vi "AO Regs Group UI.vi"(8 "error in (no error)":errorcluster, 11 "Node Ptr":T2 format="%.0x") -> (0 "error out":errorcluster)   [LabVIEW 2021, in "Modbus Master System Explorer.lvlib"]
uses:
  Modbus Master System Explorer.lvlib
  <vilib>/NI VeriStand/Custom Device API/Custom Device Item Ref.ctl
  SubVIs/Conflict Table.ctl
  SubVIs/Modbus Type.ctl
  Shared/Controls/Data Model/Mapping.ctl
  Shared/Controls/Data Model/DataType.ctl
  <vilib>/NI VeriStand/Custom Device API/Custom Device API.lvlib
  <vilib>/NI VeriStand/Custom Device Tools/Custom Device Utility Library/Custom Device Utility Library.lvlib
  Shared/Modbus Master Shared.lvlib
panel:
  in  "Delete Multiple":bool
  in  "Add One":bool
  in  "Bulk Add":bool
  out "Conflicting Holding Register Mappings":T1
  in  "Header":cluster{"Section Name":string}={"Section Name"="Holding Register Group Settings"}
  in  "Description":string
  in  "Name":string
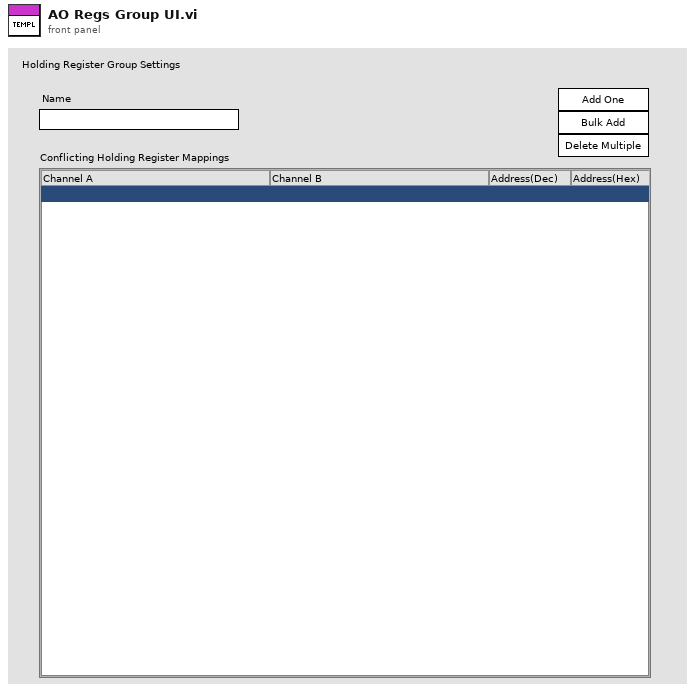
[diagram p1: front panel]
types:
  T1 = typedef "Modbus Master System Explorer.lvlib/Conflict Table.ctl" = i32
  T2 = typedef "Custom Device API.lvlib/Custom Device Item Ref.ctl" = u64
  T3 = typedef "Modbus Master Shared.lvlib/Modbus Type.ctl" = enum16{"Coil", "Discrete Input", "Holding Register", "Input Register"}
  T4 = typedef "Custom Device API.lvlib/Custom Device Item Info.ctl" = cluster{"Name":string, "Is Channel":bool, "GUID":string, "Is Waveform":bool}
  T5 = cluster{"Name":string, "Name":string, "Mapping":u16}[]
  T6 = typedef "Modbus Master Shared.lvlib/Mapping.ctl" = cluster{"DataType":T7, "Unit ID":u8, "Starting Address":u16, "Sub-Index (Bool)":u16, "VS Reference":T2}
  T7 = typedef "Modbus Master Shared.lvlib/DataType.ctl" = enum16{"Double", "Single", "I64", "I32", "I16", "I8", "U64", "U32", "U16", "U8", "Boolean"}
  T8 = typedef "Custom Device API.lvlib/Custom Device Commands.ctl" = enum16{"Default", "Item renamed", "Shutdown", "Dynamic button pressed"}
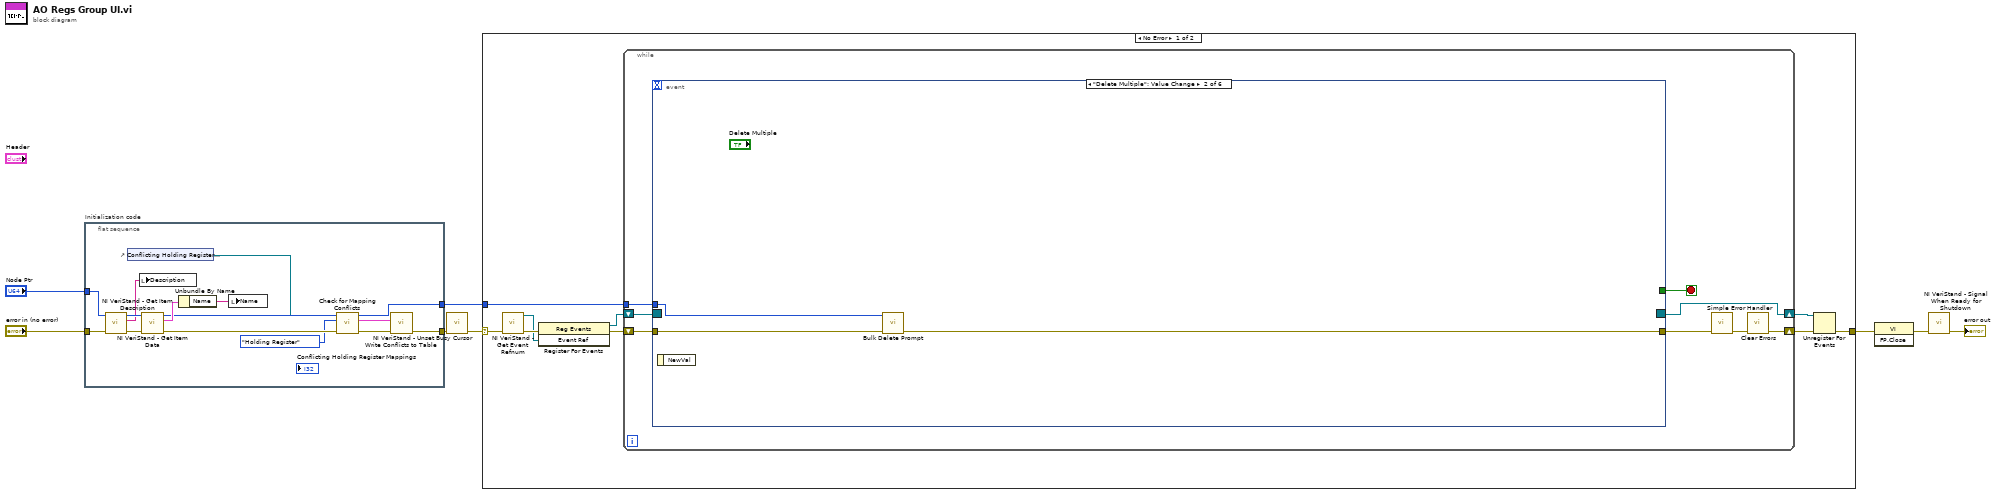
[diagram p0: block diagram]
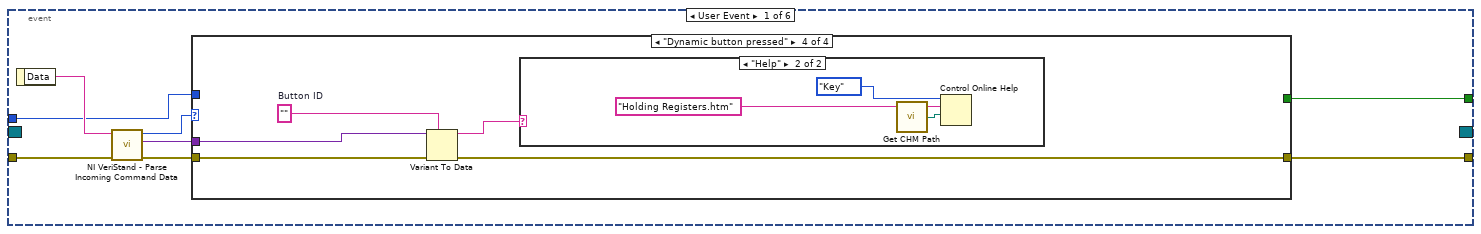
[diagram p2: hidden frame]
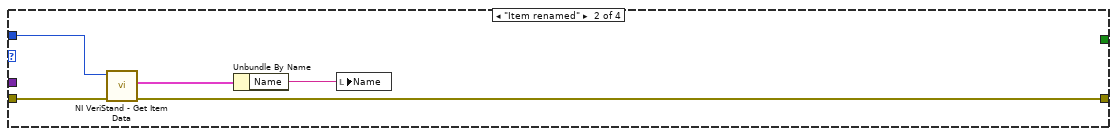
[diagram p4: hidden frame]
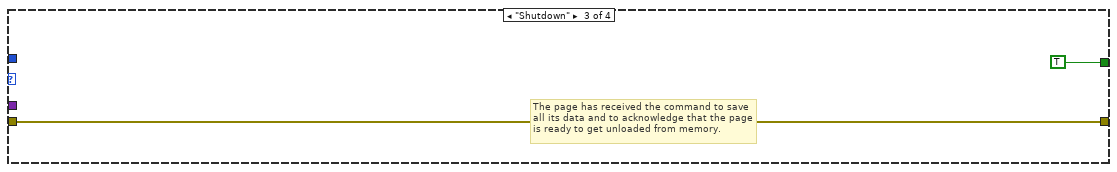
[diagram p5: hidden frame]
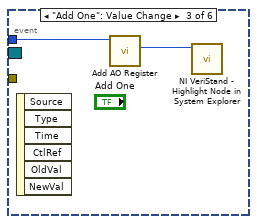
[diagram p7: hidden frame]
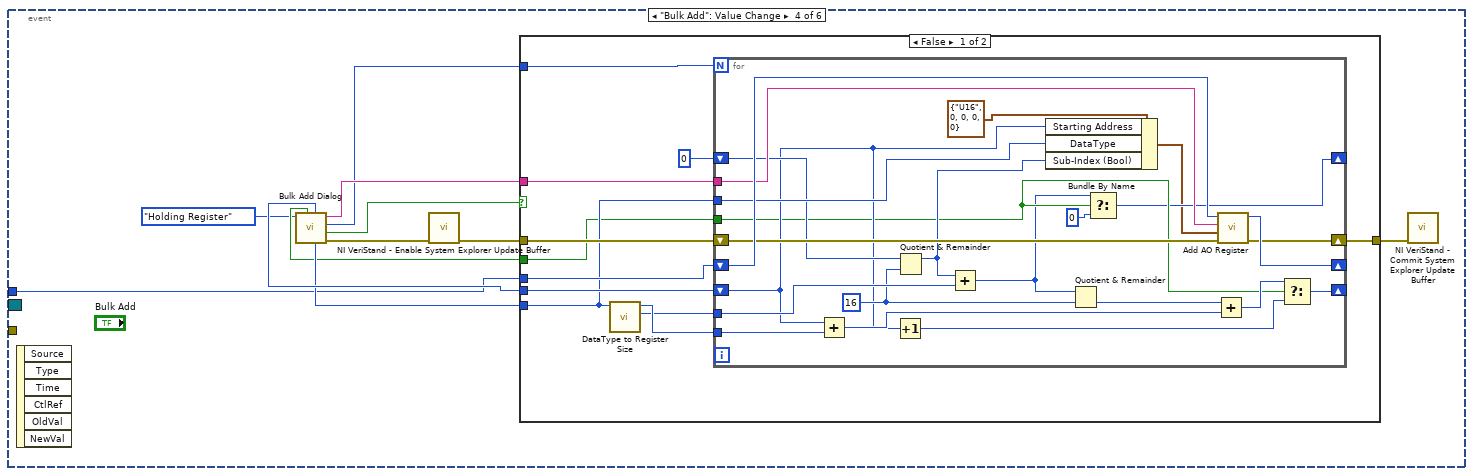
[diagram p8: hidden frame]
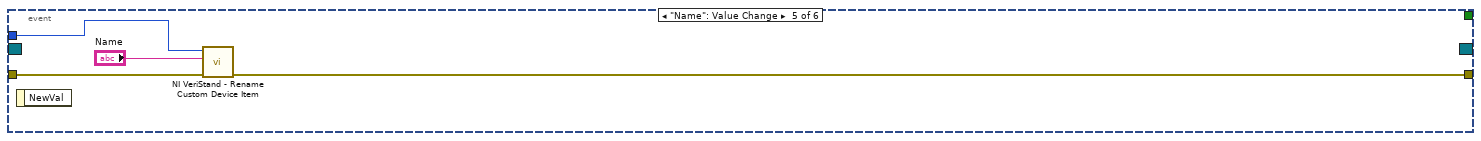
[diagram p10: hidden frame]
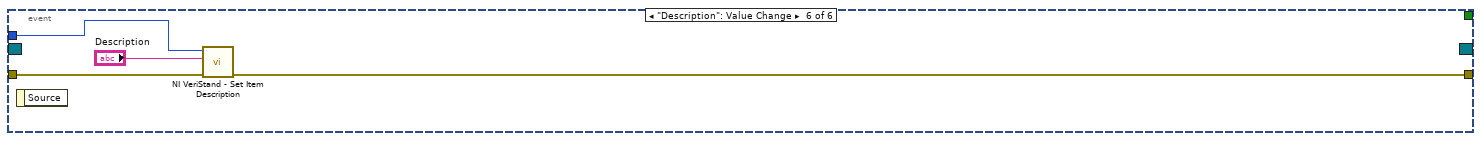
[diagram p11: hidden frame]
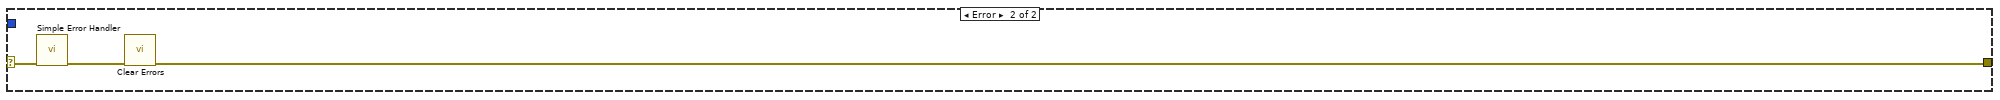
[diagram p12: hidden frame]
diagram:
  n1 = flat-sequence "Initialization code" {
    tunnel: "error in (no error)" -> [w22]
    tunnel: "Node Ptr" -> [w21]
    tunnel: [w13] -> w4
    tunnel: [w15] -> w1
    frame #0 {
      n2 = call <vilib>:"NI VeriStand - Get Item Description.vi"("error in (no error)"=w22, "Item Ref in"=w21) -> ("error out"=w19:errorcluster, "Description"=w20:string, "Item Ref out"=w23:T2)  [unwired: 7 out]
      n3 = control-ref of="Conflicting Holding Register Mappings"() -> (w10:refnum<vi>)
      n4 = local write "Description"(w20) -> ()
      n5 = call <vilib>:"NI VeriStand - Get Item Data.vi"("error in (no error)"=w19, "Item Ref in"=w23) -> ("error out"=w14:errorcluster, "Item Info"=w18:T4, "Item Ref out"=w16:T2)  [unwired: 7 out]
      n6 = Unbundle By Name(w18) -> ("Name"=w17:string)
      n7 = local write "Name"(w17) -> ()
      n8 = call "Check for Mapping Conflicts.vi"("error in (no error)"=w14, "Type"=Modbus_Type."Holding Register", "Coiil Group Ref in in"=w16) -> ("error out"=w12:errorcluster, "Array"=w11:T5, "Coiil Group Ref out"=w15:T2)  [unwired: 5 in, 1 out]
      n9 = call "Write Conflicts to Table.vi"("error in (no error)"=w12, "Conflicts"=w11, "MC Listbox Ref"=w10) -> ("error out"=w13:errorcluster)  [unwired: 8 in]
    }
  }
  n10 = call <vilib>:"NI VeriStand - Unset Busy Cursor.vi"("error in (no error)"=w4) -> ("error out"=w3:errorcluster)  [unwired: 10 out]
  n11 = case shown="No Error" w3 {
    selector: w3 -> [w24 w126]
    tunnel: [w29 w124] -> w8
    tunnel: w1 -> [w25 _]
    frame No Error {
      n12 = call <vilib>:"NI VeriStand - Get Event Refnum.vi"("error in (no error)"=w24) -> ("error out"=w32:errorcluster, "Event Ref"=w28:refnum<user-event>)  [unwired: 9 out]
      n13 = register-events(error in=w32, w28) -> (reference out=w26:refnum<event-registration>, error out=w27:errorcluster)  [unwired: 1 in]
      n14 = while {
        tunnel: w25 -> [w36]
        shift-right: [w33] -> w30
        shift-left: w27 -> [w39]
        shift-right: [w40] -> w31
        shift-left: w26 -> [w38]
        stop <- w37 stop-if-true
        n15 = event shown="[1] \"Delete Multiple\": Value Change" {
          selector: w38 -> [_ _ _ _ _ _]
          dyn-events: [_ _ _ _ _ _] -> w40
          timeout: _ -> [_ _ _ _ _ _]
          tunnel: w39 -> [w48 w66 _ _ w119 w122]
          tunnel: [w44 _ _ _ _ _] -> w37
          tunnel: [w43 w65 _ _ w118 w121] -> w35
          tunnel: w36 -> [w42 w67 w68 w70 w117 w123]
          event User Event {
            n16 = event-data() -> ("Data"=w47:string)  [unwired: 1 out]
            n17 = call <vilib>:"NI VeriStand - Parse Incoming Command Data.vi"("error in (no error)"=w48, "Incoming data"=w47) -> ("error out"=w46:errorcluster, "Outgoing data"=w41:variant, "Action"=w45:T8)  [unwired: 7 out]
            n18 = case shown="\"Dynamic button pressed\"" w45 {
              tunnel: w46 -> [w49 w54 w55 w61]
              tunnel: [_ _ TRUE _] -> w44
              tunnel: [w49 w51 w55 w58] -> w43
              tunnel: w42 -> [_ w53 _ _]
              tunnel: w41 -> [_ _ _ w60]
              frame "Default", Default {
              }
              frame "Item renamed" {
                n19 = call <vilib>:"NI VeriStand - Get Item Data.vi"("error in (no error)"=w54, "Item Ref in"=w53) -> ("error out"=w51:errorcluster, "Item Info"=w52:T4)  [unwired: 8 out]
                n20 = Unbundle By Name(w52) -> ("Name"=w50:string)
                n21 = local write "Name"(w50) -> ()
              }
              frame "Shutdown" {
                # "The page has received the command to save all its data and to acknowledge that the page is ready to get unloaded from memory."
              }
              frame "Dynamic button pressed" {
                w59 = ""  # Button ID
                n22 = Variant To Data(error in=w61, type=w59, Variant=w60) -> (data=w57:string, error out=w58:errorcluster)
                n23 = case shown="\"Help\"" w57 {
                  frame Default {
                  }
                  frame "Help" {
                    n24 = call "Get CHM Path.vi"() -> ("appended path"=w64:path)
                    n25 = Control Online Help(2:w64, 3:"Holding Registers.htm" ("String to search for"), 4:enum16{"Contents", "Key", "Close"}."Key" ("Operation")) -> ()  [unwired: 1 in, 1 out]
                  }
                }
              }
            }
          }
          event "Delete Multiple": Value Change {
            n26 = event-data() -> ()  [unwired: 2 out]
            n27 = call "Bulk Delete Prompt.vi"("error in (no error)"=w66, "Item Ref in"=w67) -> ("error out"=w65:errorcluster)  [unwired: 9 in]
          }
          event "Add One": Value Change {
            n28 = event-data() -> ()  [unwired: 7 out]
            n29 = call "Add AO Register.vi"("Node Ref In"=w68) -> ("Channel Ref out"=w69:T2)  [unwired: 8 in, 2 out]
            n30 = call <vilib>:"NI VeriStand - Highlight Node in System Explorer.vi"("Item Ref in"=w69) -> ()  [unwired: 9 in, 2 out]
          }
          event "Bulk Add": Value Change {
            n31 = event-data() -> ()  [unwired: 7 out]
            n32 = call "Bulk Add Dialog.vi"("Type"=Modbus_Type."Holding Register") -> ("error out"=w74:errorcluster, "Cancelled?"=w77:bool, "Quantity Out"=w78:u16, "Root Name Out"=w79:string, "DataType Out"=w76:T7, "Starting Address Out"=w80:u16, "Pack Values? Out"=w75:bool)  [unwired: 4 in]
            n33 = call <vilib>:"NI VeriStand - Enable System Explorer Update Buffer.vi"("error in (no error)"=w74) -> ("error out"=w73:errorcluster)  [unwired: 10 in]
            n34 = case shown="False" w77 {
              tunnel: w70 -> [w84 _]
              tunnel: w78 -> [w91 _]
              tunnel: w73 -> [w85 w115]
              tunnel: w79 -> [w90 _]
              tunnel: w80 -> [w89 _]
              tunnel: w76 -> [w83 _]
              tunnel: w75 -> [w82 _]
              tunnel: [w81 w115] -> w72
              frame False {
                n35 = call "DataType to Register Size.vi"("DataType"=w83) -> ("bits"=w86:i32, "Registers"=w88:i32)  [unwired: 9 in]
                n36 = for {
                  N: w91 -> [_]
                  shift-right: [w112] -> _
                  shift-left: w84 -> [w114]
                  shift-right: [w110] -> w81
                  shift-left: w85 -> [w113]
                  tunnel: w90 -> [w111]
                  shift-right: [w97] -> _
                  shift-left: w89 -> [w99]
                  tunnel: w83 -> [w108]
                  tunnel: w88 -> [w107]
                  shift-right: [w94] -> _
                  shift-left: 0 ("Sub-Index (Bool)") -> [w105]
                  tunnel: w86 -> [w106]
                  tunnel: w82 -> [w96]
                  w102 = 16 ("y")
                  n37 = Add(x=w99, y=w107) -> (x+y=w103:i32)
                  n38 = Increment(x=w99) -> (x+1=w100:i32)
                  n39 = Quotient & Remainder(x=w105, y=w102) -> (x-y*floor(x/y)=w104:i32)  [unwired: 1 out]
                  n40 = Add(x=w104, y=w106) -> (x+y=w95:i32)
                  n41 = Bundle By Name(cluster=T6 {"DataType"=enum."U16", "Unit ID"=0, "Starting Address"=0, "Sub-Index (Bool)"=0, "VS Reference"=0} ("Mapping"), "Starting Address"=w99, "DataType"=w108, "Sub-Index (Bool)"=w104) -> (w92:T6)
                  n42 = Quotient & Remainder(x=w95, y=w102) -> (floor(x/y)=w101:i32)  [unwired: 1 out]
                  n43 = Select(t=w95, s=w96, f=0 ("t")) -> (s? t:f=w94:i32)
                  n44 = Add(x=w101, y=w103) -> (x+y=w98:i32)
                  n45 = call "Add AO Register.vi"("error in (no error)"=w113, "Mapping"=w92, "Label"=w111, "Node Ref In"=w114) -> ("error out"=w110:errorcluster, "Node Ref out"=w112:T2)  [unwired: 5 in, 1 out]
                  n46 = Select(t=w98, s=w96, f=w100) -> (s? t:f=w97:i32)
                }
              }
              frame True {
              }
            }
            n47 = call <vilib>:"NI VeriStand - Commit System Explorer Update Buffer.vi"("error in (no error)"=w72) -> ()  [unwired: 10 in, 1 out]
          }
          event "Name": Value Change {
            n48 = event-data() -> ()  [unwired: 2 out]
            n49 = call <vilib>:"NI VeriStand - Rename Custom Device Item.vi"("error in (no error)"=w119, "New Name"="Name", "Item Ref in"=w117) -> ("error out"=w118:errorcluster)  [unwired: 1 in, 7 out]
          }
          event "Description": Value Change {
            n50 = event-data() -> ()  [unwired: 2 out]
            n51 = call <vilib>:"NI VeriStand - Set Item Description.vi"("error in (no error)"=w122, "Description"="Description", "Item Ref in"=w123) -> ("error out"=w121:errorcluster)  [unwired: 8 out]
          }
        }
        n52 = call <vilib>:"Simple Error Handler.vi"("error in (no error)"=w35) -> ("error out"=w34:errorcluster)  [unwired: 1 in, 7 out]
        n53 = call <vilib>:"Clear Errors.vi"("error in (no error)"=w34) -> ("error out"=w33:errorcluster)  [unwired: 1 in, 5 out]
      }
      n54 = Unregister For Events(event registration refnum=w31, error in=w30) -> (error out=w29:errorcluster)
    }
    frame Error {
      n55 = call <vilib>:"Simple Error Handler.vi"("error in (no error)"=w126) -> ("error out"=w125:errorcluster)  [unwired: 1 in, 7 out]
      n56 = call <vilib>:"Clear Errors.vi"("error in (no error)"=w125) -> ("error out"=w124:errorcluster)  [unwired: 1 in, 5 out]
    }
  }
  n57 = invoke class="VI" method="FP.Close"(error in=w8) -> (error out=w7:errorcluster)  [unwired: 2 in, 2 out]
  n58 = call <vilib>:"NI VeriStand - Signal When Ready for Shutdown.vi"("error in (no error)"=w7) -> ("error out"=→"error out":errorcluster)  [unwired: 10 out]
